vi "Configure Basic PID Parameters.vi"(0 "VISA resource name":refnum<visa-resource-name>, 1 "Unit Address (1)":u8=1, 5 "PID Number  (1)":u8=1 min=1 max=3, 7 "Proportional Band (0)":i32, 9 "Integral Time (0)":i32, 11 "error in (no error)":errorcluster, 12 "Derivative Time (0)":i32) -> (4 "VISA resource name out":refnum<visa-resource-name>, 15 "error out":errorcluster)   [LabVIEW 2014, in "Eurotherm 35xx Series.lvlib"]
doc: "This VI sets basic PID parameters."
uses:
  <instrlib>/Eurotherm 35xx Series/Eurotherm 35xx Series.lvlib
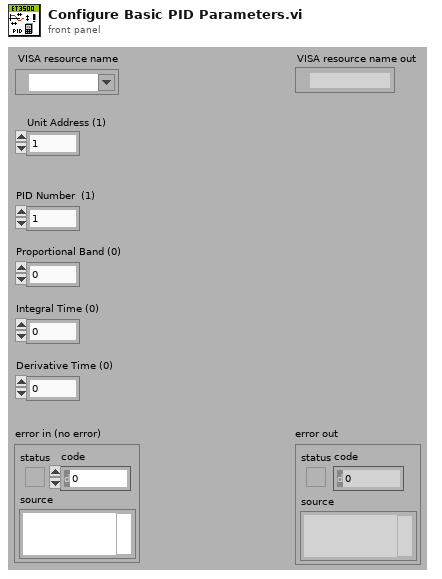
[diagram p1: front panel]
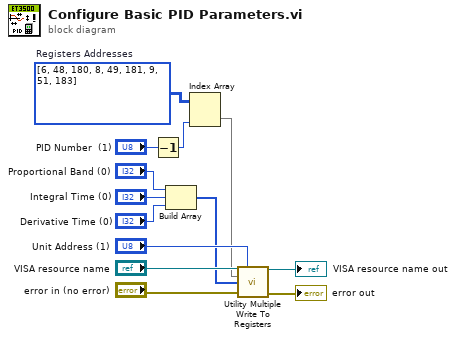
[diagram p0: block diagram]
diagram:
  w13 = u16[][] [[6, 48, 180], [8, 49, 181], [9, 51, 183]]  # Registers Addresses
  n1 = Decrement(x="PID Number  (1)") -> (x-1=w11:u8)
  n2 = Build Array("Proportional Band (0)", "Integral Time (0)", "Derivative Time (0)") -> (w1:i32[])
  n3 = Index Array(array=w13, index (col)=w11) -> (element=w2:u16[])  [unwired: 1 in]
  n4 = call <instrlib>:"Utility Multiple Write To Registers.vi"("VISA resource name"="VISA resource name", "Unit Address (1)"="Unit Address (1)", "Registers Addresses (0)"=w2, "Data (0)"=w1, "error in (no error)"="error in (no error)") -> ("VISA resource name out"=→"VISA resource name out":refnum<visa-resource-name>, "error out"=→"error out":errorcluster)  [unwired: 9 in]
